vi "SortContour.vi"(11 "LineArray":T4[](array[typedef])) -> (3 "Polys":T2[](array[typedef]))   [LabVIEW 2014]
uses:
  TypeDefs/Line2D.ctl
  TypeDefs/Point2D.ctl
  TypeDefs/Poly2D.ctl
panel:
  out "XY Graph":T1(graph)
  out "SizeEnd":i32
  out "sorted array":T2[](array[typedef])
  out "SizeStart":i32
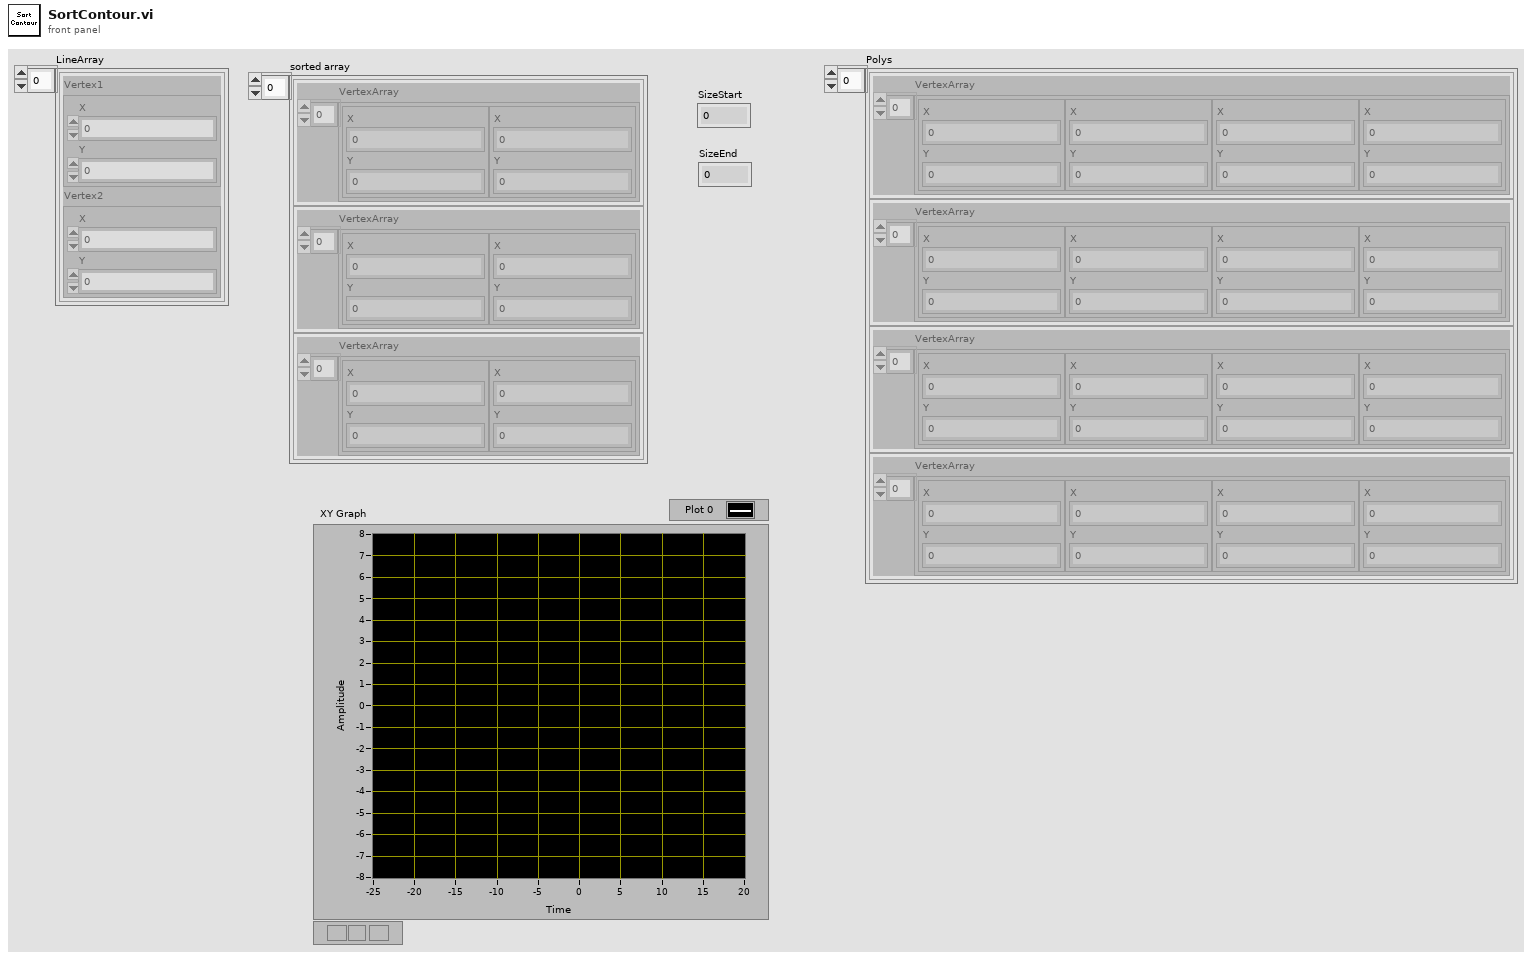
[diagram p1: front panel]
types:
  T1 = cluster{"VertexArray":cluster{"X":sgl, "Y":sgl}[]}[]
  T2 = typedef "Poly2D.ctl" = cluster{"VertexArray":T3[]}
  T3 = typedef "Point2D.ctl" = cluster{"X":sgl, "Y":sgl}
  T4 = typedef "Line2D.ctl" = cluster{"Vertex1":T3, "Vertex2":T3}
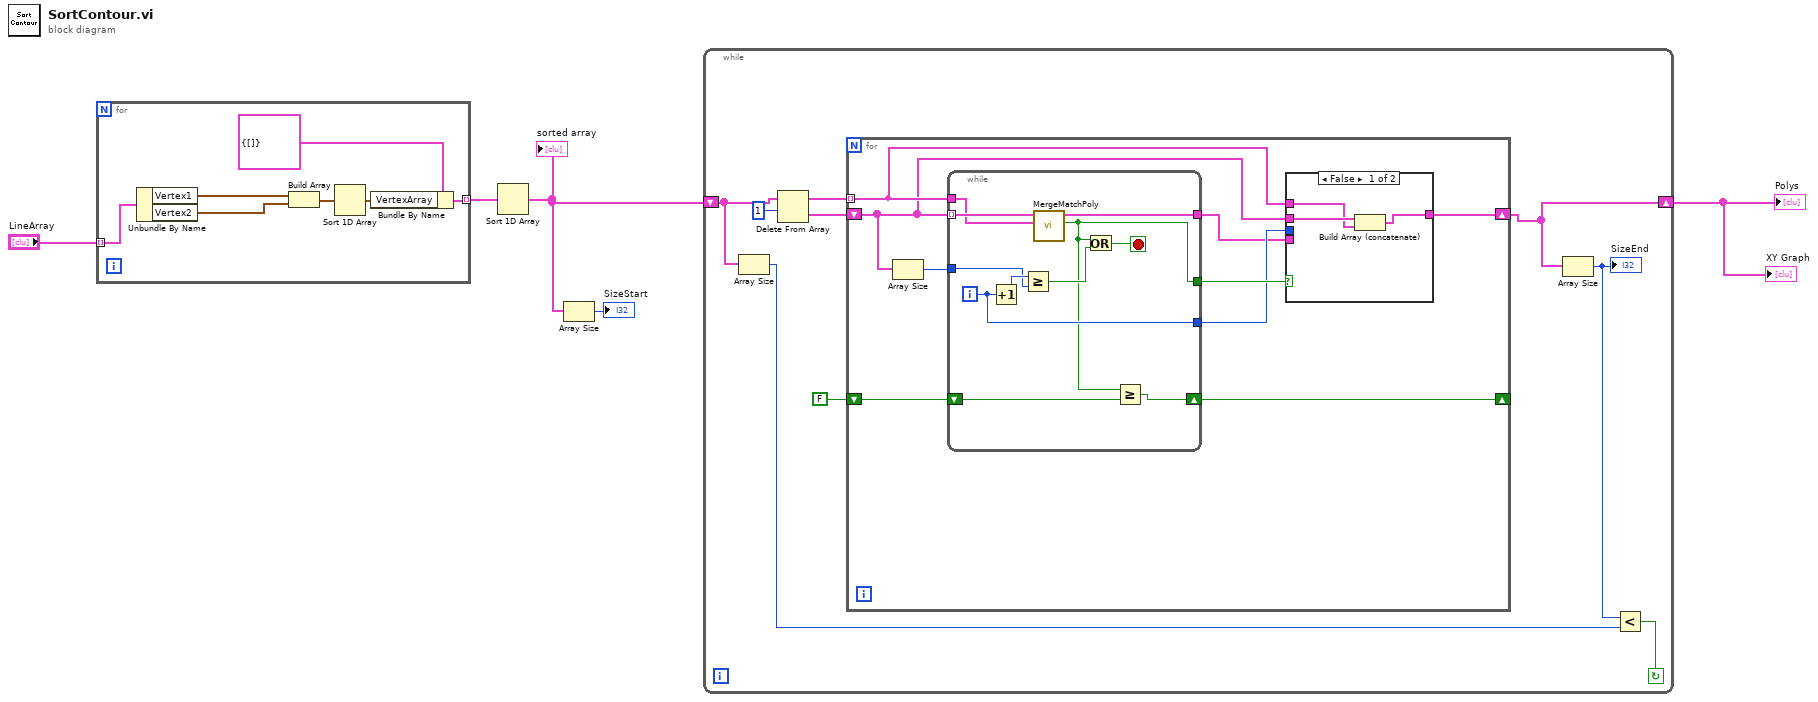
[diagram p0: block diagram]
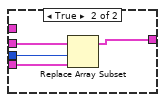
[diagram p2: hidden frame]
diagram:
  n1 = for {
    tunnel: "LineArray" -> [w12] mode=indexing
    tunnel: [w6] -> w4 mode=indexing
    n2 = Unbundle By Name(w12) -> ("Vertex1"=w11:T3, "Vertex2"=w10:T3)
    n3 = Build Array(w11, w10) -> (w9:T3[])
    n4 = Sort 1D Array(array=w9) -> (sorted array=w7:T3[])
    n5 = Bundle By Name(cluster=T2 {"VertexArray"=[]} ("Poly2D"), "VertexArray"=w7) -> (w6:T2)
  }
  n6 = Sort 1D Array(array=w4) -> (sorted array=w2:T2[])
  "sorted array" <- w2
  n7 = Array Size(array=w2) -> (size(s)=→"SizeStart":i32)
  n8 = while {
    shift-right: [w21] -> w1
    shift-left: w2 -> [w16]
    stop <- w13 continue-if-true
    n9 = Array Size(array=w16) -> (size(s)=w14:i32)
    n10 = Delete From Array(array=w16, length=1) -> (deleted portion=w18:T2[], array with subset deleted=w19:T2[])  [unwired: 1 in]
    n11 = for {
      tunnel: w19 -> [w25] mode=indexing
      shift-right: [w26] -> w21
      shift-left: w18 -> [w24]
      shift-right: [w22] -> _
      shift-left: FALSE -> [w23]
      n12 = Array Size(array=w24) -> (size(s)=w30:i32)
      n13 = while {
        tunnel: w25 -> [w47]
        tunnel: w24 -> [w48] mode=indexing
        tunnel: w30 -> [w45]
        tunnel: [w43] -> w27
        tunnel: [w42] -> w28
        tunnel: [w40] -> w29
        shift-right: [w38] -> w22
        shift-left: w23 -> [w39]
        i -> [w42]
        stop <- w44 stop-if-true
        n14 = Increment(x=w42) -> (x+1=w46:i32)
        n15 = Greater Or Equal?(x=w46, y=w45) -> (x >= y?=w41:bool)
        n16 = call "MergeMatchPoly.vi"("Poly2D_2"=w47, "Poly2D_1"=w48) -> ("Matched"=w40:bool, "Poly2D"=w43:T2)  [unwired: 8 in]
        n17 = Or(x=w40, y=w41) -> (x .or. y?=w44:bool)
        n18 = Greater Or Equal?(x=w40, y=w39) -> (x >= y?=w38:bool)
      }
      n19 = case shown="False" w29 {
        tunnel: w24 -> [w33 w37]
        tunnel: w28 -> [_ w36]
        tunnel: w27 -> [_ w35]
        tunnel: [w31 w34] -> w26
        tunnel: w25 -> [w32 _]
        frame False {
          n20 = Build Array (concatenate)(w33, w32) -> (w31:T2[])
        }
        frame True {
          n21 = Replace Array Subset(array=w37, new element=w35, index=w36) -> (w34:T2[])
        }
      }
    }
    n22 = Array Size(array=w21) -> (size(s)=w15:i32)
    "SizeEnd" <- w15
    n23 = Less?(x=w15, y=w14) -> (x < y?=w13:bool)
  }
  "Polys" <- w1
  "XY Graph" <- w1
